vi "toDistance.vi"(0 "height of camera off ground IN":dbl, 1 "angle from zero camera DEGREES":dbl, 2 "angle from fov to target IN":dbl) -> (7 "distance to target IN":dbl)   [LabVIEW 2020]
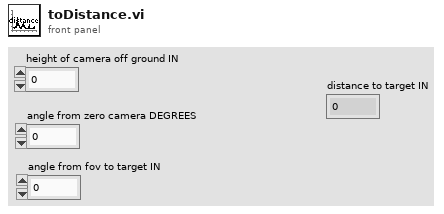
[diagram p1: front panel]
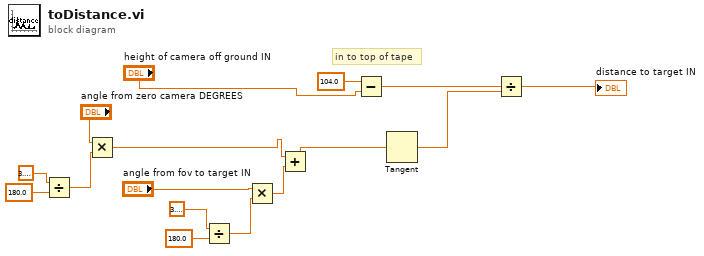
[diagram p0: block diagram]
diagram:
  # "in to top of tape"
  n1 = Divide(x=3.141592653589793, y=180.0) -> (x/y=w5:dbl)
  n2 = Multiply(x="angle from zero camera DEGREES", y=w5) -> (x*y=w4:dbl)
  n3 = Divide(x=3.141592653589793, y=180.0) -> (x/y=w7:dbl)
  n4 = Multiply(x="angle from fov to target IN", y=w7) -> (x*y=w10:dbl)
  n5 = Add(x=w4, y=w10) -> (x+y=w12:dbl)
  n6 = Subtract(x=104.0, y="height of camera off ground IN") -> (x-y=w14:dbl)
  n7 = Tangent(1:w12) -> (0:w13:dbl)
  n8 = Divide(x=w14, y=w13) -> (x/y=→"distance to target IN":dbl)
